vi "scan_system_red.vi"(8 "error in":errorcluster, 11 "address":string) -> (0 "error out":errorcluster)   [LabVIEW 2020]
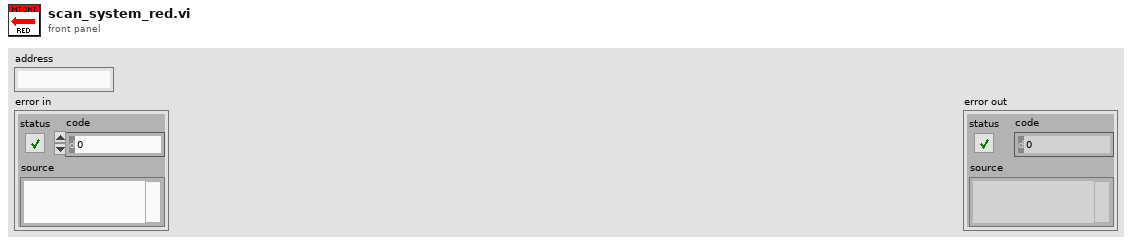
[diagram p1: front panel]
types:
  T1 = enum16{"Standard", "Buffered", "CRLF", "Immediate"}
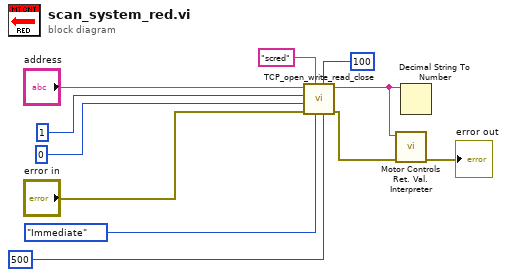
[diagram p0: block diagram]
diagram:
  n1 = call "TCP_open_write_read_close.vi"("timeout ms (25000)"=500, "bytes to read"=100, "mode (standard)"=T1."Immediate", "write string"="scred", "error in"="error in", "local port (0)"=u16 0, "remote port or service name"=u16 1, "address"="address") -> ("error out"=w5:errorcluster, "read string"=w3:string)  [unwired: 2 in]
  n2 = call "Motor Controls Ret. Val. Interpreter.vi"("error in"=w5, "Command Return"=w3) -> ("error out"=→"error out":errorcluster)  [unwired: 8 in, 1 out]
  n3 = Decimal String To Number(string=w3) -> ()  [unwired: 2 in, 2 out]
